vi "TrajectoryCommonTuning.vi"() -> (1 "out POSe":T7 {"ROTATION"."SIN" format="%13.4f"; "ROTATION"."COS" format="%13.4f"; "ROTATION"."VALUE" format="%13.4f"; "TRANSLATION"."Y" format="%14.3f"; "TRANSLATION"."X" format="%14.3f"}, 3 "HOLONOMIC_CTRL_PACK_TUNING":T1 {"thetaProfiledPID_CTRL"."Constraint"."MaxAcceleration" format="%16_6e"; "thetaProfiledPID_CTRL"."Constraint"."MaxVelocity" format="%16_6e"; "thetaProfiledPID_CTRL"."Setpoint"."Velocity" format="%16_6e"; "thetaProfiledPID_CTRL"."Setpoint"."Position" format="%16_6e"; "thetaProfiledPID_CTRL"."Goal"."Velocity" format="%16_6e"; "thetaProfiledPID_CTRL"."Goal"."Position" format="%16_6e"; "thetaProfiledPID_CTRL"."Controller"."IntegralZone" format="%16_6e"; "thetaProfiledPID_CTRL"."Controller"."Measurement" format="%16_6e"; "thetaProfiledPID_CTRL"."Controller"."Prev_F_P_2" format="%16_6e"; "thetaProfiledPID_CTRL"."Controller"."Prev_F_P" format="%16_6e"; "thetaProfiledPID_CTRL"."Controller"."Max_Output" format="%16_6e"; "thetaProfiledPID_CTRL"."Controller"."Min_Output" format="%16_6e"; "thetaProfiledPID_CTRL"."Controller"."Prev_Deriv 2" format="%16_6e"; "thetaProfiledPID_CTRL"."Controller"."Prev_Deriv" format="%16_6e"; "thetaProfiledPID_CTRL"."Controller"."Kf" format="%16_6e"; "thetaProfiledPID_CTRL"."Controller"."SetPoint" format="%16_6e"; "thetaProfiledPID_CTRL"."Controller"."VelocityTolerance" format="%16_6e"; "thetaProfiledPID_CTRL"."Controller"."PositionTolerance" format="%16_6e"; "thetaProfiledPID_CTRL"."Controller"."Total_Integral" format="%16_6e"; "thetaProfiledPID_CTRL"."Controller"."PrevError" format="%16_6e"; "thetaProfiledPID_CTRL"."Controller"."VelocityError" format="%16_6e"; "thetaProfiledPID_CTRL"."Controller"."PositionError" format="%16_6e"; "thetaProfiledPID_CTRL"."Controller"."Min_Input" format="%16_6e"; "thetaProfiledPID_CTRL"."Controller"."Max_Input" format="%16_6e"; "thetaProfiledPID_CTRL"."Controller"."Min_Integral" format="%16_6e"; "thetaProfiledPID_CTRL"."Controller"."Max_Integral" format="%16_6e"; "thetaProfiledPID_CTRL"."Controller"."Period" format="%16_6e"; "thetaProfiledPID_CTRL"."Controller"."Kd" format="%16_6e"; "thetaProfiledPID_CTRL"."Controller"."Ki" format="%16_6e"; "thetaProfiledPID_CTRL"."Controller"."Kp" format="%16_6e"})   [LabVIEW 2023]
uses:
  <vilib>/Rock Robotics/WPI/ThirdParty/JAS_Junk/TrajLib/TypeDef/POSE2D.ctl
  <vilib>/Rock Robotics/WPI/ThirdParty/JAS_Junk/TrajLib/TypeDef/TRANSLATION2D.ctl
  <vilib>/Rock Robotics/WPI/ThirdParty/JAS_Junk/TrajLib/TypeDef/ROTATION2D.ctl
  <vilib>/Rock Robotics/WPI/ThirdParty/JAS_Junk/TrajLib/TypeDef/HOLONOMIC_PACK_TUNING.ctl
  <vilib>/Rock Robotics/WPI/ThirdParty/JAS_Junk/TrajLib/TypeDef/PID_TUNING.ctl
  <vilib>/Rock Robotics/WPI/ThirdParty/JAS_Junk/TrajLib/TypeDef/PROFILED_PID_CONTROLLER.ctl
  <vilib>/Rock Robotics/WPI/ThirdParty/JAS_Junk/TrajLib/TypeDef/PID_CONTROLLER.ctl
  <vilib>/Rock Robotics/WPI/ThirdParty/JAS_Junk/TrajLib/TypeDef/TRAPEZOID_PROFILE_STATE.ctl
  <vilib>/Rock Robotics/WPI/ThirdParty/JAS_Junk/TrajLib/TypeDef/TRAPEZOID_PROFILE_CONSTRAINT.ctl
  <vilib>/Rock Robotics/WPI/ThirdParty/JAS_Junk/TrajLib/ProfiledPIDController_NewPeriod.vi
  <vilib>/Rock Robotics/WPI/ThirdParty/JAS_Junk/TrajLib/ProfiledPIDController_SetIntegratorRange.vi
  <vilib>/Rock Robotics/WPI/ThirdParty/JAS_Junk/TrajLib/ProfiledPIDController_DisableContInput.vi
  <vilib>/Rock Robotics/WPI/ThirdParty/JAS_Junk/TrajLib/ProfiledPIDController_EnableContInput.vi
  <vilib>/Rock Robotics/WPI/ThirdParty/JAS_Junk/TrajLib/TrapProfConstraint_New.vi
  <vilib>/Rock Robotics/WPI/ThirdParty/JAS_Junk/TrajLib/Rotation2d_CreateAngle.vi
  <vilib>/Rock Robotics/WPI/ThirdParty/JAS_Junk/TrajLib/Translation2d_Create.vi
  <vilib>/Rock Robotics/WPI/ThirdParty/JAS_Junk/TrajLib/TrapProfState_New.vi
  <vilib>/Rock Robotics/WPI/ThirdParty/JAS_Junk/TrajLib/PIDController_NewPeriod.vi
  <vilib>/Rock Robotics/SystemInterfaces/NetworkCommunication/NetComm_UsageReport_report.vi
  <vilib>/Rock Robotics/WPI/ThirdParty/JAS_Junk/TrajLib/PIDController_SetIntegratorRange.vi
  <vilib>/Rock Robotics/WPI/ThirdParty/JAS_Junk/TrajLib/PIDController_DisableContinousInput.vi
  <vilib>/Rock Robotics/WPI/ThirdParty/JAS_Junk/TrajLib/PIDController_EnableContinousInput.vi
  <vilib>/Rock Robotics/WPI/ThirdParty/JAS_Junk/TrajLib/Globals/Util_LibraryGlobals.vi
  <vilib>/Rock Robotics/WPI/ThirdParty/JAS_Junk/TrajLib/Trajectory_Library.lvlib
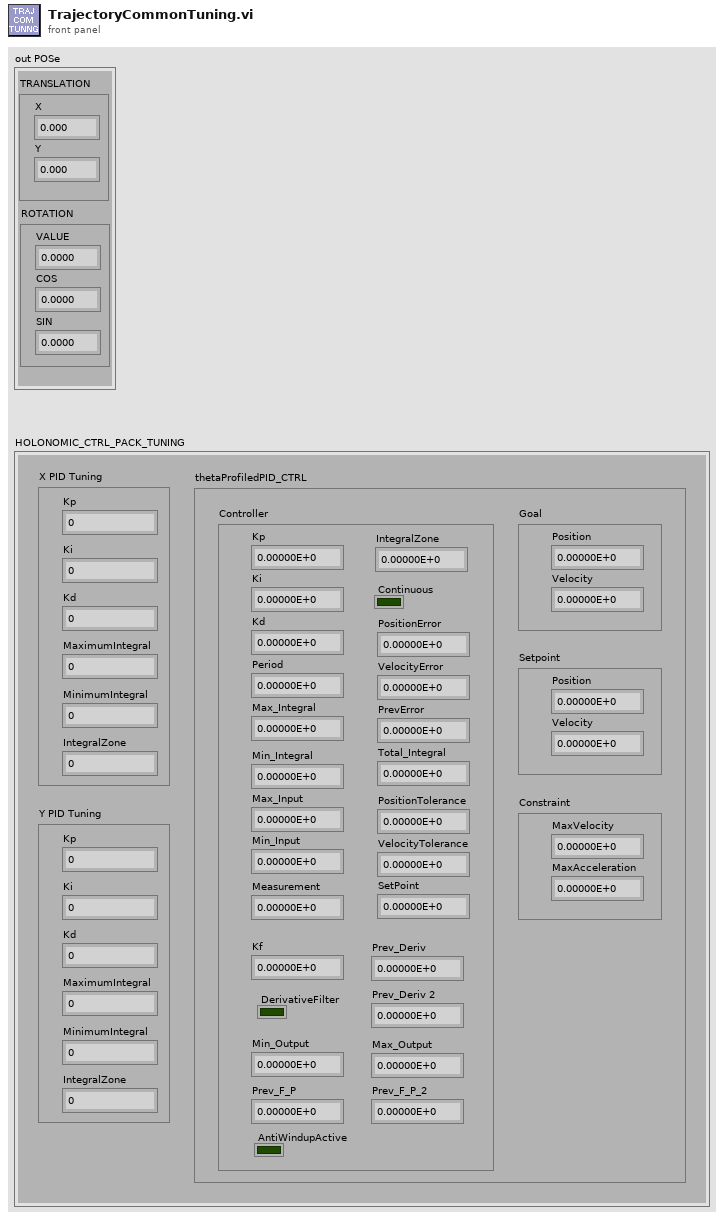
[diagram p1: front panel]
types:
  T1 = typedef "Trajectory_Library.lvlib/HOLONOMIC_PACK_TUNING.ctl" = cluster{"X PID Tuning":T2, "Y PID Tuning":T2, "thetaProfiledPID_CTRL":T3}
  T2 = typedef "Trajectory_Library.lvlib/PID_TUNING.ctl" = cluster{"Kp":dbl, "Ki":dbl, "Kd":dbl, "MaximumIntegral":dbl, "MinimumIntegral":dbl, "IntegralZone":dbl}
  T3 = typedef "Trajectory_Library.lvlib/PROFILED_PID_CONTROLLER.ctl" = cluster{"Controller":T4, "Goal":T5, "Setpoint":T5, "Constraint":T6}
  T4 = typedef "Trajectory_Library.lvlib/PID_CONTROLLER.ctl" = cluster{"Kp":dbl, "Ki":dbl, "Kd":dbl, "Period":dbl, "Max_Integral":dbl, "Min_Integral":dbl, "Max_Input":dbl, "Min_Input":dbl, "Continuous":bool, "PositionError":dbl, "VelocityError":dbl, "PrevError":dbl, "Total_Integral":dbl, "PositionTolerance":dbl, "VelocityTolerance":dbl, "SetPoint":dbl, "Kf":dbl, "Prev_Deriv":dbl, "Prev_Deriv 2":dbl, "DerivativeFilter":bool, "Min_Output":dbl, "Max_Output":dbl, "Prev_F_P":dbl, "Prev_F_P_2":dbl, "AntiWindupActive":bool, "Measurement":dbl, "IntegralZone":dbl}
  T5 = typedef "Trajectory_Library.lvlib/TRAPEZOID_PROFILE_STATE.ctl" = cluster{"Position":dbl, "Velocity":dbl}
  T6 = typedef "Trajectory_Library.lvlib/TRAPEZOID_PROFILE_CONSTRAINT.ctl" = cluster{"MaxVelocity":dbl, "MaxAcceleration":dbl}
  T7 = typedef "Trajectory_Library.lvlib/POSE2D.ctl" = cluster{"TRANSLATION":T8, "ROTATION":T9}
  T8 = typedef "Trajectory_Library.lvlib/TRANSLATION2D.ctl" = cluster{"X":dbl, "Y":dbl}
  T9 = typedef "Trajectory_Library.lvlib/ROTATION2D.ctl" = cluster{"VALUE":dbl, "COS":dbl, "SIN":dbl}
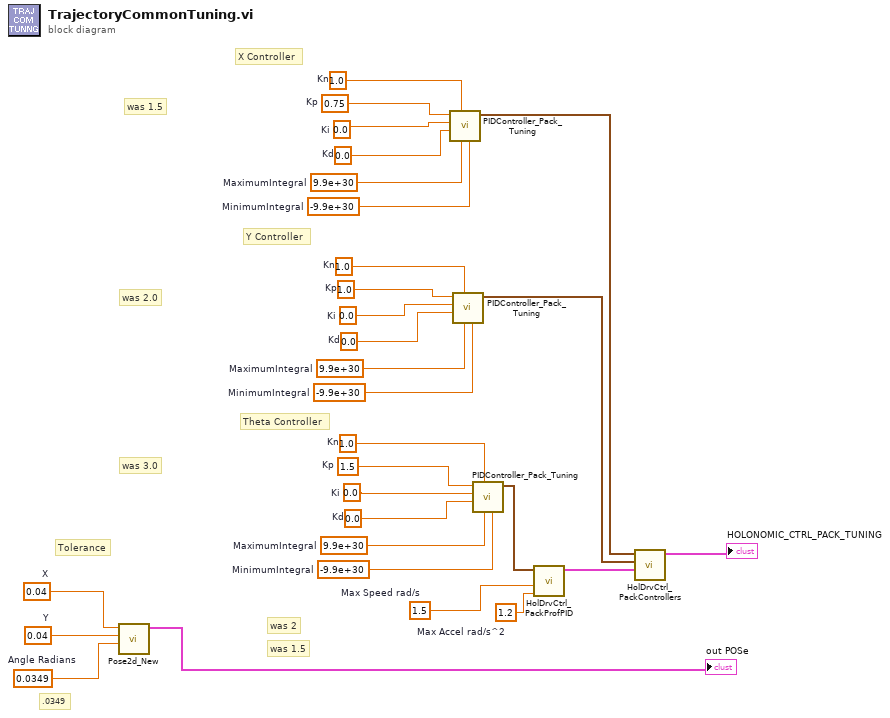
[diagram p0: block diagram]
diagram:
  w27 = 0.04  # X
  w28 = 0.04  # Y
  w26 = 0.0349  # Angle Radians
  w25 = 1.2  # Max Accel rad/s^2
  w24 = 1.5  # Max Speed rad/s
  w20 = 1.0  # Kn
  w17 = 1.5  # Kp
  w8 = 0.0  # Ki
  w7 = 0.0  # Kd
  w6 = 9.9e+30  # MaximumIntegral
  w5 = -9.9e+30  # MinimumIntegral
  w22 = 1.0  # Kn
  w19 = 0.75  # Kp
  w16 = 0.0  # Ki
  w15 = 0.0  # Kd
  w14 = 9.9e+30  # MaximumIntegral
  w13 = -9.9e+30  # MinimumIntegral
  w21 = 1.0  # Kn
  w18 = 1.0  # Kp
  w12 = 0.0  # Ki
  w11 = 0.0  # Kd
  w10 = 9.9e+30  # MaximumIntegral
  w9 = -9.9e+30  # MinimumIntegral
  # "was 1.5"
  # "was 2"
  # "was 3.0"
  # "was 2.0"
  # "was 1.5"
  # ".0349"
  # "Tolerance"
  # "Theta Controller"
  # "Y Controller"
  # "X Controller"
  n1 = call <vilib>:"Pose2d_New.vi"("Heading"=w26, "Y"=w28, "X"=w27) -> ("out POSe"=→"out POSe":T7)  [unwired: 8 in]
  n2 = call <vilib>:"PIDController_Pack_Tuning.vi"("MinimumIntegral"=w13, "MaximumIntegral"=w14, "Kn"=w22, "Kd"=w15, "Ki"=w16, "Kp"=w19) -> ("PID Tuning"=w4:T2)  [unwired: 5 in]
  n3 = call <vilib>:"PIDController_Pack_Tuning.vi"("MinimumIntegral"=w9, "MaximumIntegral"=w10, "Kn"=w21, "Kd"=w11, "Ki"=w12, "Kp"=w18) -> ("PID Tuning"=w3:T2)  [unwired: 5 in]
  n4 = call <vilib>:"PIDController_Pack_Tuning.vi"("MinimumIntegral"=w5, "MaximumIntegral"=w6, "Kn"=w20, "Kd"=w7, "Ki"=w8, "Kp"=w17) -> ("PID Tuning"=w23:T2)  [unwired: 5 in]
  n5 = call <vilib>:"HolDrvCtrl_PackProfPID.vi"("Max Accel"=w25, "Max Speed"=w24, "Theta PID Tuning"=w23) -> ("Theta PID CONTROLLER"=w2:T3)  [unwired: 8 in]
  n6 = call <vilib>:"HolDrvCtrl_PackControllers.vi"("thetaProfiledPID_CTRL"=w2, "Y PID Tuning"=w3, "X PID Tuning"=w4) -> ("HOLONOMIC_CTRL_PACK_TUNING"=→"HOLONOMIC_CTRL_PACK_TUNING":T1)  [unwired: 8 in]
